vi "Write Preview.vi"(10 "Preview?":bool, 11 "SolutionBuilder in":refnum<class "SolutionBuilder.lvclass">) -> (3 "SolutionBuilder out":refnum<class "SolutionBuilder.lvclass">)   [LabVIEW 2019, in "SolutionBuilder.lvlib" / "SolutionBuilder.lvclass"]
uses:
  SolutionBuilder.lvclass
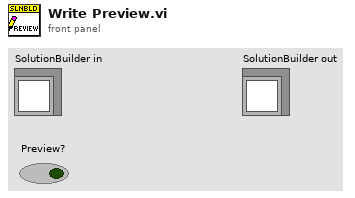
[diagram p1: front panel]
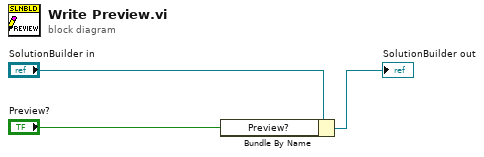
[diagram p0: block diagram]
diagram:
  n1 = Bundle By Name(cluster="SolutionBuilder in", "Preview?"="Preview?") -> (→"SolutionBuilder out":refnum<class "SolutionBuilder.lvclass">)
